vi "Drive Control Loop.vi"() -> ()   [LabVIEW 2019]
uses:
  Calculations or utilities/Is command done typedef.ctl
  <vilib>/Rock Robotics/WPI/ThirdParty/Phoenix-LabVIEW/Motor Controller/Controls/CTRE_Phoenix_MotorControl_ControlMode.ctl
  <vilib>/Rock Robotics/WPI/ThirdParty/Phoenix-LabVIEW/Pigeon IMU/CTRE_PigeonIMU_GetYPR.vi
  <vilib>/Rock Robotics/Network Tables/NT Read Number.vi
  <vilib>/addons/control/pid/pid.llb/PID (DBL).vi
  Drive Global.vi
  <vilib>/addons/control/pid/NI_PID_pid.lvlib
panel:
  in  "max speed (u/100ms)":dbl
  in  "Auto-align acceptable error (deg)":dbl=1.0
  in  "Turning PID gains":T1={"proportional gain"=1.0, "integral gain"=0.01, "derivative gain"=0.0} {"derivative gain" format="%.3f"; "integral gain" format="%.3f"; "proportional gain" format="%.3f"}
  in  "Acceptable turning Error (deg)":dbl=1.0
  out "Gyro (deg)":dbl(graph)
  out "Drive Velocity (u/100ms)":T2(graph)
  out "Drive Position (ft)":T3(graph)
  in  "Acceptable Position Error (ft)":dbl
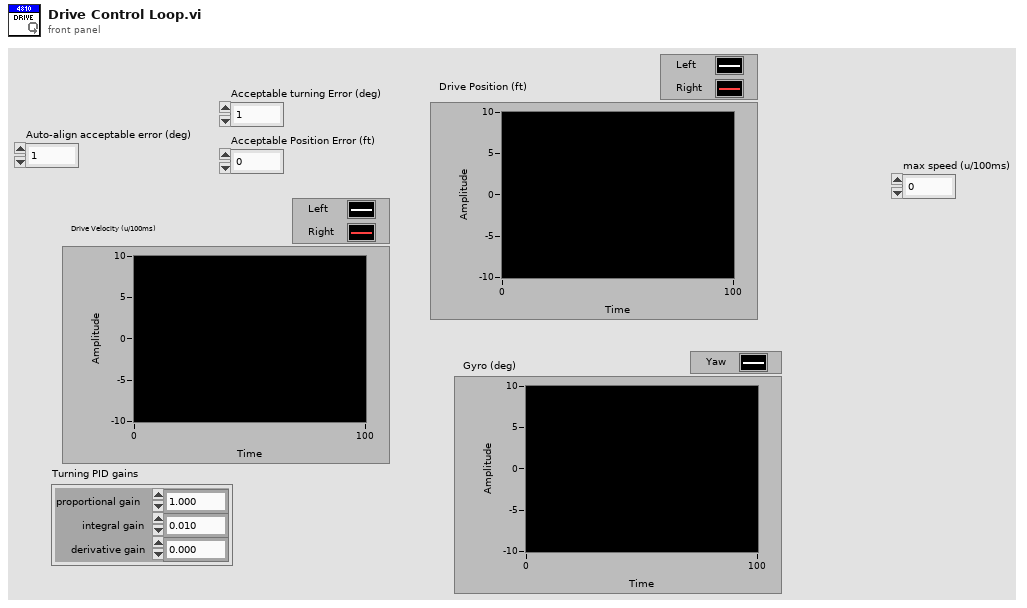
[diagram p1: front panel]
types:
  T1 = cluster{"proportional gain":dbl, "integral gain":dbl, "derivative gain":dbl}
  T2 = cluster{"Left Velocity (u/100ms)":i32, "Right Velocity (u/100ms)":i32}
  T3 = cluster{"Drive Position out (ft)":dbl, "Drive Position out (ft)":dbl}
  T4 = typedef "CTRE_PigeonIMU_DeviceRef.ctl" = cluster{"DeviceStatus":errorcluster, "Device Number":u8, "Type":T5, "Device ID":u32, "Handle":u64, "UsageFrame":u32, "Library Path":path}
  T5 = typedef "CTRE_PigeonIMU_ConnectionType.ctl" = u32
  T6 = typedef "WPI_MotorControlDeviceRef.ctl" = cluster{"DeviceStatus":errorcluster, "Type":T7, "PWM":cluster{"PWM Channel":T8, "DeadBand":T9}, "CAN":cluster{"Device Number":u8, "SetOutput VI Ref":variant, "GetOutput VI Ref":variant, "Enable VI Ref":variant, "Disable VI Ref":variant, "Data":variant}, "Invert":bool, "DIO PWM":cluster{"PWM \"Enable\" Channel":T8, "DIOChannel":T10, "PWM Rate":dbl}}
  T7 = typedef "WPI_MotorControlType.ctl" = enum16{"PWM", "CAN", "DIO PWM"}
  T8 = typedef "FPGA_DIOPWMChannel.ctl" = enum8{"PWM 0", "PWM 1", "PWM 2", "PWM 3", "PWM 4", "PWM 5", "PWM 6", "PWM 7", "PWM 8", "PWM 9", "PWM MXP 0", "PWM MXP 1", "PWM MXP 2", "PWM MXP 3", "PWM MXP 4", "PWM MXP 5", "PWM MXP 6", "PWM MXP 7", "PWM MXP 8", "PWM MXP 9", "Invalid"}
  T9 = typedef "WPI_PWMDeadband.ctl" = cluster{"Name":string, "maxPositivePwm":i32, "minPositivePwm":i32, "centerPwm":i32, "maxNegativePwm":i32, "minNegativePwm":i32, "angularRange":u16}
  T10 = typedef "FPGA_DIOChannel.ctl" = enum8{"DIO 0", "DIO 1", "DIO 2", "DIO 3", "DIO 4", "DIO 5", "DIO 6", "DIO 7", "DIO 8", "DIO 9", "DIO MXP 0", "DIO MXP 1", "DIO MXP 2", "DIO MXP 3", "DIO MXP 4", "DIO MXP 5", "DIO MXP 6", "DIO MXP 7", "DIO MXP 8", "DIO MXP 9", "DIO MXP 10", "DIO MXP 11", "DIO MXP 12", "DIO MXP 13", "DIO MXP 14", "DIO MXP 15", "SPI Port CS1", "SPI Port CS2", "SPI Port CS3", "SPI Port MISO", "SPI Port MOSI", "Invalid"}
  T11 = typedef "Is command done typedef.ctl" = cluster{"Done?":bool, "Timestamp [ms]":dbl}
  T12 = typedef "Drive Command Typedef.ctl" = cluster{"Drive Mode":T13, "LeftValue(%)/ relative Distance[ft]":dbl, "Right Motor Value(%)/ absolute angle (deg)":dbl, "Timestamp (ms)":dbl}
  T13 = typedef "Drive Mode Typedef.ctl" = enum16{"Disabled", "Auto-align", "Drive Distance", "Turn to angle", "Driver", "Driver Velocity Control"}
  T14 = typedef "CTRE_Phoenix_MotorControl_ControlMode.ctl" = u16
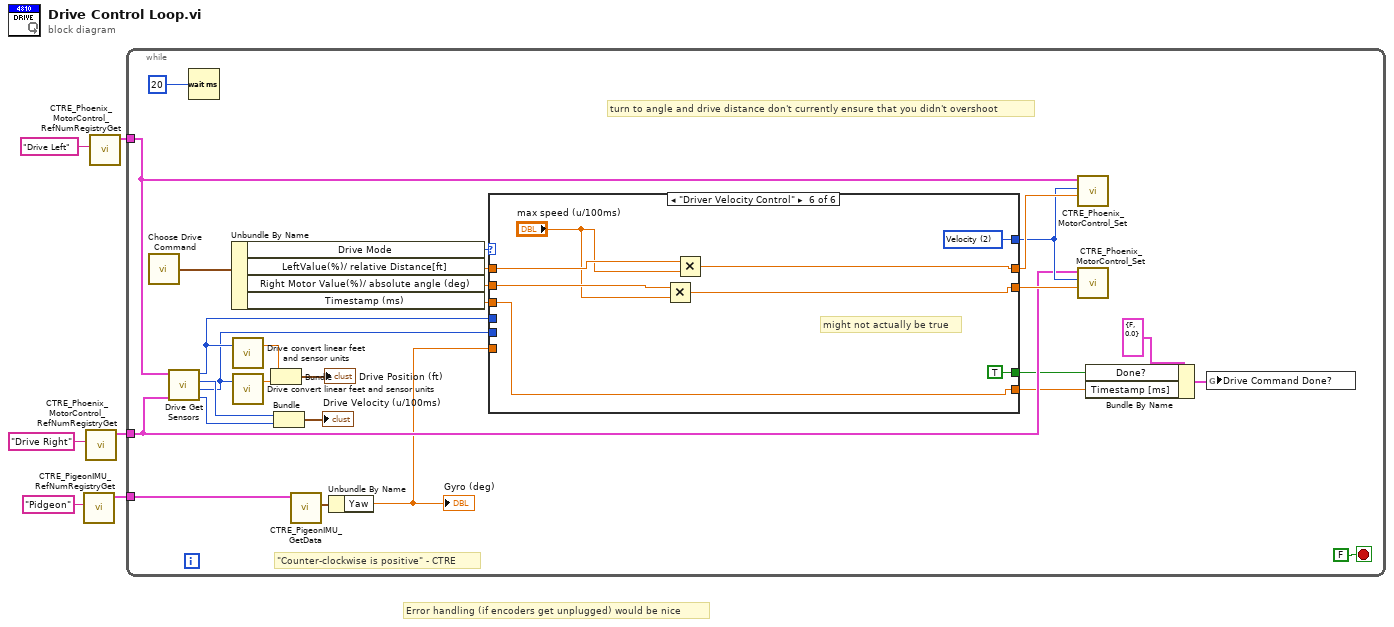
[diagram p0: block diagram]
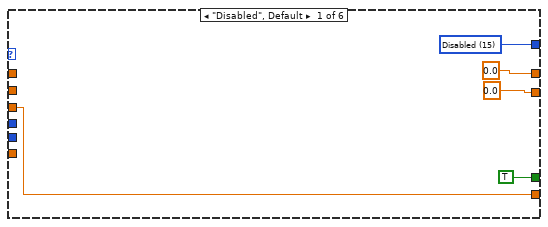
[diagram p2: hidden frame]
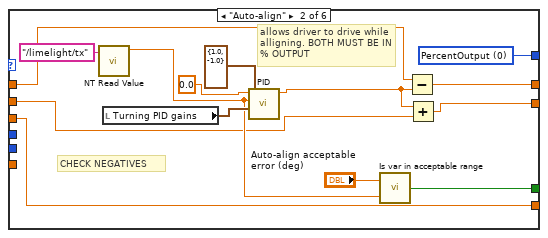
[diagram p3: hidden frame]
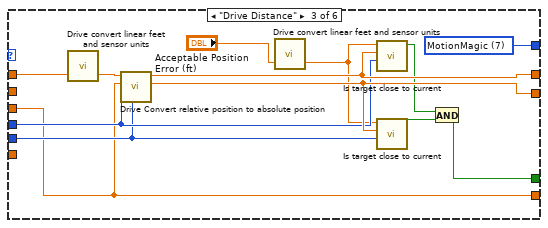
[diagram p4: hidden frame]
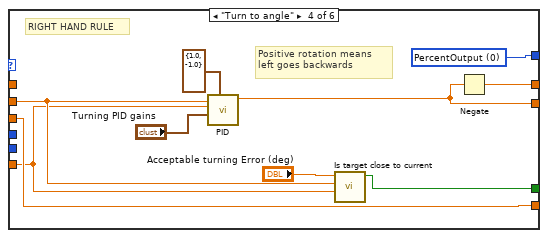
[diagram p5: hidden frame]
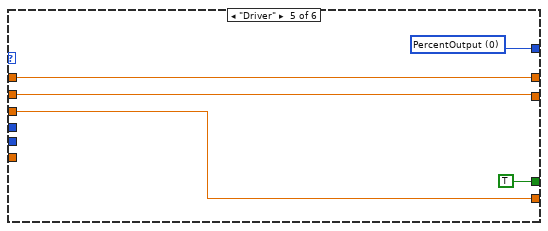
[diagram p6: hidden frame]
diagram:
  # "Error handling (if encoders get unplugged) would be nice"
  n1 = call <vilib>:"CTRE_PigeonIMU_RefNumRegistryGet.vi"("refnum name"="Pidgeon") -> ("PigeonIMUDevRef"=w1:T4)  [unwired: 9 in, 1 out]
  n2 = call <vilib>:"CTRE_Phoenix_MotorControl_RefNumRegistryGet.vi"("refnum name"="Drive Right") -> ("PhoenixMotorControlDevRef"=w3:T6)  [unwired: 9 in, 1 out]
  n3 = call <vilib>:"CTRE_Phoenix_MotorControl_RefNumRegistryGet.vi"("refnum name"="Drive Left") -> ("PhoenixMotorControlDevRef"=w4:T6)  [unwired: 9 in, 1 out]
  n4 = while {
    tunnel: w4 -> [w25]
    tunnel: w3 -> [w24]
    tunnel: w1 -> [w14]
    stop <- FALSE stop-if-true
    # "\"Counter-clockwise is positive\" - CTRE"
    # "turn to angle and drive distance don't currently ensure that you didn't overshoot"
    n5 = call "Choose Drive Command.vi"() -> ("Current Drive Command"=w27:T12)  [unwired: 1 in]
    n6 = call "Drive Get Sensors.vi"("Right Drive DevRef"=w24, "Left Drive DevRef"=w25) -> ("Right Velocity (u/100ms)"=w22:i32, "Right Position (u)"=w7:i32, "Left Velocity (u/100ms)"=w23:i32, "Left Position (u)"=w9:i32)  [unwired: 6 in]
    n7 = Wait (ms)(milliseconds to wait=u32 20) -> ()  [unwired: 1 out]
    n8 = Unbundle By Name(w27) -> ("Drive Mode"=w31:T13, "LeftValue(%)/ relative Distance[ft]"=w18:dbl, "Right Motor Value(%)/ absolute angle (deg)"=w17:dbl, "Timestamp (ms)"=w16:dbl)
    n9 = call "Drive convert linear feet and sensor units.vi"("Drive position in (u)"=w9) -> ("Drive Position out (ft)"=w10:dbl)  [unwired: 1 in, 1 out]
    n10 = call "Drive convert linear feet and sensor units.vi"("Drive position in (u)"=w7) -> ("Drive Position out (ft)"=w8:dbl)  [unwired: 1 in, 1 out]
    n11 = Bundle("Drive Position out (ft)"=w10, "Drive Position out (ft)"=w8) -> (→"Drive Position (ft)":T3)  [unwired: 1 in]
    n12 = Bundle("Left Velocity (u/100ms)"=w23, "Right Velocity (u/100ms)"=w22) -> (→"Drive Velocity (u/100ms)":T2)  [unwired: 1 in]
    n13 = call-poly <vilib>:"CTRE_PigeonIMU_GetData.vi"("PigeonIMUDevRef"=w14) -> ("Yaw Pitch Roll"=w13:cluster{"Yaw":dbl, "Pitch":dbl, "Roll":dbl})  [unwired: 8 in, 2 out]
    n14 = Unbundle By Name(w13) -> ("Yaw"=w12:dbl)
    "Gyro (deg)" <- w12
    n15 = case shown="\"Driver Velocity Control\"" w31 {
      tunnel: [w38 w51 w65 w75 w80 w88] -> w28
      tunnel: [0.0 ("Output") w39 w64 w67 w78 w84] -> w30
      tunnel: [0.0 ("Output") w40 w63 w66 w77 w83] -> w29
      tunnel: w9 -> [_ _ w59 _ _ _]
      tunnel: w7 -> [_ _ w58 _ _ _]
      tunnel: [TRUE w46 w60 w72 TRUE TRUE ("Acceptable")] -> w19
      tunnel: w18 -> [_ w43 w56 _ w78 w87]
      tunnel: w17 -> [_ w41 _ w71 w77 w86]
      tunnel: [w34 w52 w55 w74 w76 w82] -> w15
      tunnel: w16 -> [w34 w52 w55 w74 w76 w82]
      tunnel: w12 -> [_ _ _ w70 _ _]
      frame "Disabled", Default {
        w38 = T14 15 items=["PercentOutput"=0, "Position"=1, "Velocity"=2, "Current"=3, "Follower"=5, "MotionProfile"=6, "MotionMagic"=7, "MotionProfileArc"=10, "Disabled"=15] ("Control Mode")
      }
      frame "Auto-align" {
        w51 = T14 0 items=["PercentOutput"=0, "Position"=1, "Velocity"=2, "Current"=3, "Follower"=5, "MotionProfile"=6, "MotionMagic"=7, "MotionProfileArc"=10, "Disabled"=15] ("Control Mode")
        # "allows driver to drive while alligning. BOTH MUST BE IN % OUTPUT"
        # "CHECK NEGATIVES"
        n16 = call-poly <vilib>:"NT Read Value.vi"("Name"="/limelight/tx") -> ("Numeric"=w45:dbl)  [unwired: 9 in, 1 out]
        n17 = local read "Turning PID gains"() -> (w49:T1)
        n18 = call-poly <vilib>:"PID.vi"("output range"=cluster{"output high":dbl, "output low":dbl} {"output high"=1.0, "output low"=-1.0}, "PID gains"=w49, "process variable"=w45, "setpoint"=0.0 ("dt (s)")) -> ("output"=w42:dbl)  [unwired: 6 in, 1 out]
        n19 = call "Is var in acceptable range.vi"("Variable"=w45, "Acceptable plus minus"="Auto-align acceptable error (deg)") -> ("Acceptable"=w46:bool)
        n20 = Subtract(x=w43, y=w42) -> (x-y=w39:dbl)
        n21 = Add(x=w42, y=w41) -> (x+y=w40:dbl)
      }
      frame "Drive Distance" {
        w65 = T14 7 items=["PercentOutput"=0, "Position"=1, "Velocity"=2, "Current"=3, "Follower"=5, "MotionProfile"=6, "MotionMagic"=7, "MotionProfileArc"=10, "Disabled"=15] ("Control Mode")
        n22 = call "Drive convert linear feet and sensor units.vi"("Drive position in (feet)"=w56) -> ("Drive Position out (u)"=w57:dbl)  [unwired: 1 in, 1 out]
        n23 = call "Drive Convert relative position to absolute position.vi"("Right Encoder position"=w58, "Left Encoder Position"=w59, "Timestamp [ms]"=w55, "Relative Distance change"=w57) -> ("Right Target Position"=w63:dbl, "Left Target Position"=w64:dbl)  [unwired: 6 in]
        n24 = call "Drive convert linear feet and sensor units.vi"("Drive position in (feet)"="Acceptable Position Error (ft)") -> ("Drive Position out (u)"=w53:dbl)  [unwired: 1 in, 1 out]
        n25 = call "Is target close to current.vi"("Current Position"=w59, "Target Position"=w64, "Acceptable Error"=w53) -> ("Acceptable"=w61:bool)  [unwired: 8 in]
        n26 = call "Is target close to current.vi"("Current Position"=w58, "Target Position"=w63, "Acceptable Error"=w53) -> ("Acceptable"=w62:bool)  [unwired: 8 in]
        n27 = And(x=w61, y=w62) -> (x .and. y?=w60:bool)
      }
      frame "Turn to angle" {
        w75 = T14 0 items=["PercentOutput"=0, "Position"=1, "Velocity"=2, "Current"=3, "Follower"=5, "MotionProfile"=6, "MotionMagic"=7, "MotionProfileArc"=10, "Disabled"=15] ("Control Mode")
        # "Positive rotation means left goes backwards"
        # "RIGHT HAND RULE"
        n28 = call-poly <vilib>:"PID.vi"("output range"=cluster{"output high":dbl, "output low":dbl} {"output high"=1.0, "output low"=-1.0}, "PID gains"="Turning PID gains", "process variable"=w70, "setpoint"=w71) -> ("output"=w66:dbl)  [unwired: 6 in, 1 out]
        n29 = call "Is target close to current.vi"("Current Position"=w70, "Target Position"=w71, "Acceptable Error"="Acceptable turning Error (deg)") -> ("Acceptable"=w72:bool)  [unwired: 8 in]
        n30 = Negate(x=w66) -> (-x=w67:dbl)
      }
      frame "Driver" {
        w80 = T14 0 items=["PercentOutput"=0, "Position"=1, "Velocity"=2, "Current"=3, "Follower"=5, "MotionProfile"=6, "MotionMagic"=7, "MotionProfileArc"=10, "Disabled"=15] ("Control Mode")
      }
      frame "Driver Velocity Control" {
        w88 = T14 2 items=["PercentOutput"=0, "Position"=1, "Velocity"=2, "Current"=3, "Follower"=5, "MotionProfile"=6, "MotionMagic"=7, "MotionProfileArc"=10, "Disabled"=15] ("Control Mode")
        # "might not actually be true"
        n31 = Multiply(x=w86, y="max speed (u/100ms)") -> (x*y=w83:dbl)
        n32 = Multiply(x=w87, y="max speed (u/100ms)") -> (x*y=w84:dbl)
      }
    }
    n33 = call <vilib>:"CTRE_Phoenix_MotorControl_Set.vi"("Output"=w30, "Control Mode"=w28, "PhoenixMotorControlDevRef"=w25) -> ()  [unwired: 7 in, 2 out]
    n34 = call <vilib>:"CTRE_Phoenix_MotorControl_Set.vi"("Output"=w29, "Control Mode"=w28, "PhoenixMotorControlDevRef"=w24) -> ()  [unwired: 7 in, 2 out]
    n35 = Bundle By Name(cluster=T11 {"Done?"=FALSE, "Timestamp [ms]"=0.0} ("Command Done?"), "Done?"=w19, "Timestamp [ms]"=w15) -> (w11:T11)
    n36 = global write "Drive Global.vi" "Drive Command Done?"(w11) -> ()
  }
